vi "Parse Single Item.vi"(7 "Quoted String? (F)":bool, 11 "String In":string) -> (2 "Remaining":string, 3 "Item":string, 5 "JSON Item Type":T1=enum."null")   [LabVIEW 2020, in "JSON.lvlib"]
uses:
  JSON.lvlib
  JSON Item Type.ctl
  Unescape String.vi
  <vilib>/regexp/Match Regular Expression.xnode
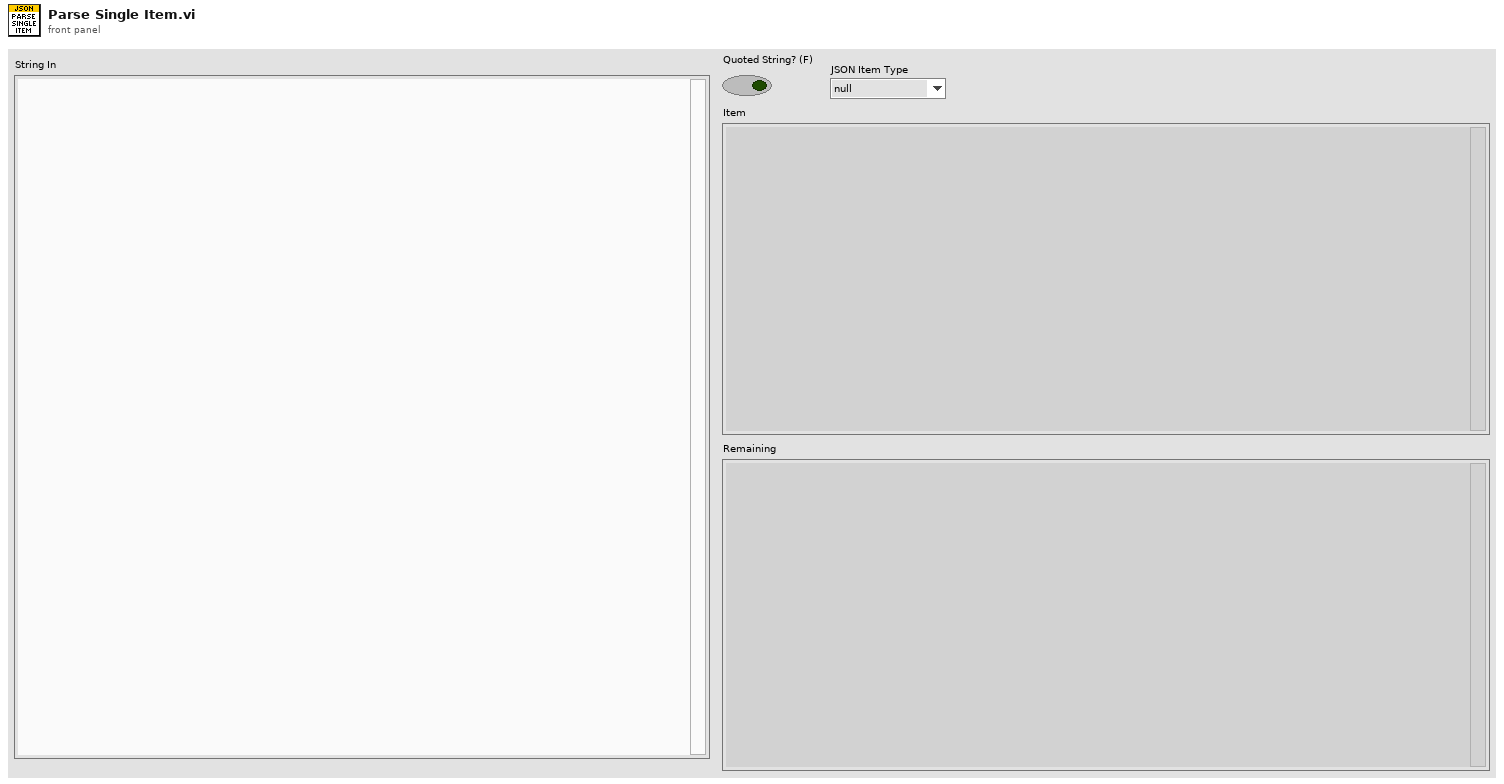
[diagram p1: front panel]
types:
  T1 = typedef "JSON.lvlib/JSON Item Type.ctl" = enum16{"unknown", "null", "Array", "Object", "String", "Number", "Boolean"}
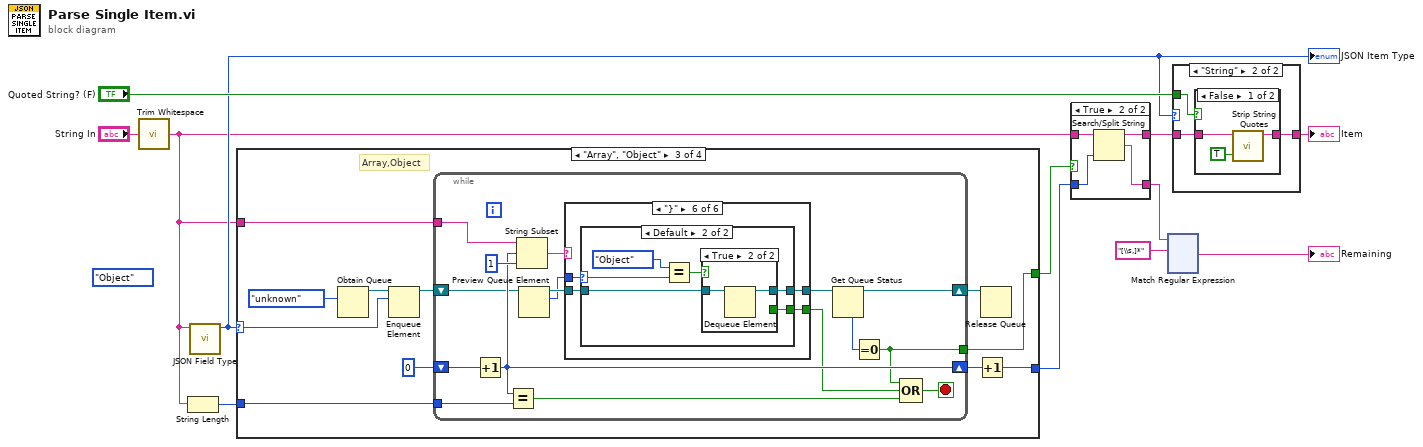
[diagram p0: block diagram]
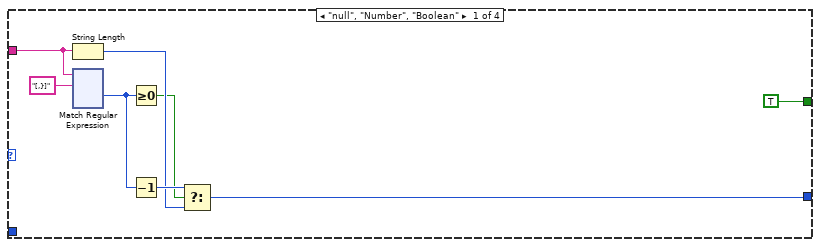
[diagram p4: hidden frame]
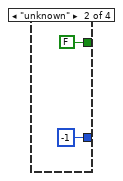
[diagram p5: hidden frame]
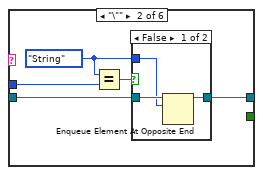
[diagram p7: hidden frame]
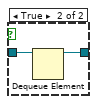
[diagram p8: hidden frame]
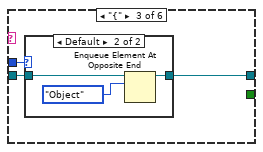
[diagram p9: hidden frame]
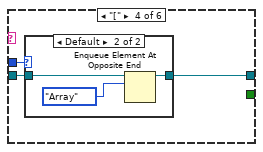
[diagram p11: hidden frame]
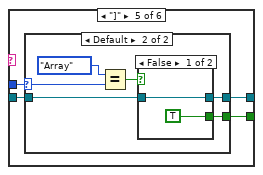
[diagram p13: hidden frame]
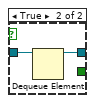
[diagram p15: hidden frame]
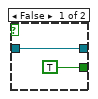
[diagram p17: hidden frame]
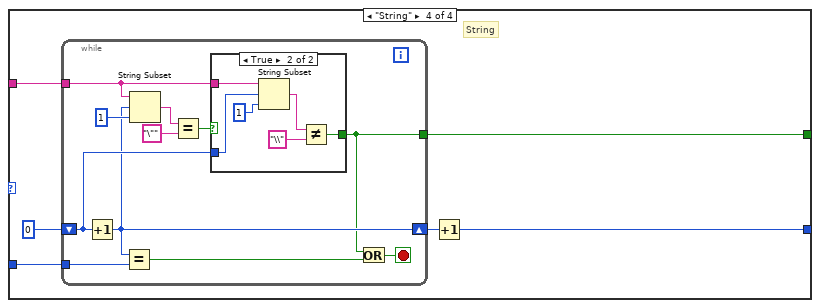
[diagram p18: hidden frame]
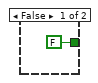
[diagram p19: hidden frame]
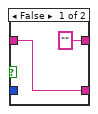
[diagram p20: hidden frame]
diagram:
  (unwired) JSON_Item_Type."Object" ("JSON Item Type")
  n1 = call <vilib>:"Trim Whitespace.vi"("string"="String In") -> ("trimmed string"=w1:string)  [unwired: 1 in]
  n2 = String Length(string=w1) -> (length=w11:i32)
  n3 = call "JSON Field Type.vi"("JSON String"=w1) -> ("JSON Item Type"=w2:T1)  [unwired: 10 in]
  "JSON Item Type" <- w2
  n4 = case shown="\"String\"" w2 {
    selector: w2 -> [_ _ w146 _]
    tunnel: w1 -> [w18 _ w144 w224]
    tunnel: w11 -> [_ _ w142 w223]
    tunnel: [w13 -1 w139 w219] -> w10
    tunnel: [TRUE FALSE w141 w220] -> w9
    frame "null", "Number", "Boolean" {
      n5 = String Length(string=w18) -> (length=w16:i32)
      n6 = xnode "Match Regular Expression"("input string"=w18, "regular expression"="[,}]") -> ("offset past match"=w19:i32)  [unwired: 4 in, 4 out]
      n7 = Greater Or Equal To 0?(x=w19) -> (x >= 0?=w15:bool)
      n8 = Decrement(x=w19) -> (x-1=w17:i32)
      n9 = Select(t=w17, s=w15, f=w16) -> (s? t:f=w13:i32)
    }
    frame "unknown" {
    }
    frame "Array", "Object" {
      # "Array,Object"
      n10 = Obtain Queue(element data type=JSON_Item_Type."unknown" ("JSON Item Type")) -> (queue out=w147:refnum<queue>)  [unwired: 4 in, 2 out]
      n11 = Enqueue Element(queue=w147, element=w146) -> (queue out=w145:refnum<queue>)  [unwired: 2 in, 2 out]
      n12 = while {
        shift-right: [w150] -> w138
        shift-left: w145 -> [w155]
        tunnel: w144 -> [w160]
        shift-right: [w156] -> w140
        shift-left: 0 -> [w158]
        tunnel: w142 -> [w163]
        tunnel: [w148] -> w141
        stop <- w161 stop-if-true
        n13 = Increment(x=w158) -> (x+1=w156:i32)
        n14 = Equal?(x=w156, y=w163) -> (x = y?=w162:bool)
        n15 = String Subset(string=w160, offset (0)=w156, length (rest)=1 ("length (rest)")) -> (substring=w157:string)
        n16 = Preview Queue Element(queue=w155) -> (queue out=w154:refnum<queue>, element=w153:T1)  [unwired: 2 in, 2 out]
        n17 = case shown="\"}\"" w157 {
          tunnel: w153 -> [_ w168 w175 w182 w190 w205]
          tunnel: w154 -> [w164 w167 w177 w184 w192 w207]
          tunnel: [w164 w166 w176 w183 w191 w206] -> w151
          tunnel: [_ _ _ _ w189 w204] -> w152
          frame Default {
          }
          frame "\"" {
            w165 = JSON_Item_Type."String" ("JSON Item Type")
            n18 = Equal?(x=w165, y=w168) -> (x = y?=w169:bool)
            n19 = case shown="False" w169 {
              tunnel: w167 -> [w172 w174]
              tunnel: [w171 w173] -> w166
              tunnel: w165 -> [w170 _]
              frame False {
                n20 = Enqueue Element At Opposite End(queue=w172, element=w170) -> (queue out=w171:refnum<queue>)  [unwired: 2 in, 2 out]
              }
              frame True {
                n21 = Dequeue Element(queue=w174) -> (queue out=w173:refnum<queue>)  [unwired: 2 in, 3 out]
              }
            }
          }
          frame "{" {
            n22 = case shown="Default" w175 {
              tunnel: w177 -> [w178 w181]
              tunnel: [w178 w180] -> w176
              frame "String" {
              }
              frame Default {
                n23 = Enqueue Element At Opposite End(queue=w181, element=JSON_Item_Type."Object" ("JSON Item Type")) -> (queue out=w180:refnum<queue>)  [unwired: 2 in, 2 out]
              }
            }
          }
          frame "[" {
            n24 = case shown="Default" w182 {
              tunnel: w184 -> [w185 w188]
              tunnel: [w185 w187] -> w183
              frame "String" {
              }
              frame Default {
                n25 = Enqueue Element At Opposite End(queue=w188, element=JSON_Item_Type."Array" ("JSON Item Type")) -> (queue out=w187:refnum<queue>)  [unwired: 2 in, 2 out]
              }
            }
          }
          frame "]" {
            n26 = case shown="Default" w190 {
              selector: w190 -> [_ w199]
              tunnel: w192 -> [w193 w197]
              tunnel: [w193 w196] -> w191
              tunnel: [_ w195] -> w189
              frame "String" {
              }
              frame Default {
                n27 = Equal?(x=JSON_Item_Type."Array" ("JSON Item Type"), y=w199) -> (x = y?=w198:bool)
                n28 = case shown="False" w198 {
                  tunnel: w197 -> [w201 w203]
                  tunnel: [w201 w202] -> w196
                  tunnel: [TRUE _] -> w195
                  frame False {
                  }
                  frame True {
                    n29 = Dequeue Element(queue=w203) -> (queue out=w202:refnum<queue>)  [unwired: 2 in, 3 out]
                  }
                }
              }
            }
          }
          frame "}" {
            n30 = case shown="Default" w205 {
              selector: w205 -> [_ w214]
              tunnel: w207 -> [w208 w212]
              tunnel: [w208 w211] -> w206
              tunnel: [_ w210] -> w204
              frame "String" {
              }
              frame Default {
                n31 = Equal?(x=JSON_Item_Type."Object" ("JSON Item Type"), y=w214) -> (x = y?=w213:bool)
                n32 = case shown="True" w213 {
                  tunnel: w212 -> [w216 w218]
                  tunnel: [w216 w217] -> w211
                  tunnel: [TRUE _] -> w210
                  frame False {
                  }
                  frame True {
                    n33 = Dequeue Element(queue=w218) -> (queue out=w217:refnum<queue>)  [unwired: 2 in, 3 out]
                  }
                }
              }
            }
          }
        }
        n34 = Get Queue Status(queue=w151) -> (queue out=w150:refnum<queue>, # elements in queue=w149:i32)  [unwired: 2 in, 6 out]
        n35 = Equal To 0?(x=w149) -> (x = 0?=w148:bool)
        n36 = Compound Arithmetic op=OR(w148, w152, w162) -> (w161:bool)
      }
      n37 = Increment(x=w140) -> (x+1=w139:i32)
      n38 = Release Queue(queue=w138) -> ()  [unwired: 2 in, 3 out]
    }
    frame "String" {
      # "String"
      n39 = while {
        tunnel: w224 -> [w229]
        shift-right: [w227] -> w221
        shift-left: 0 ("length (rest)") -> [w228]
        tunnel: w223 -> [w235]
        tunnel: [w226] -> w220
        stop <- w234 stop-if-true
        n40 = Increment(x=w228) -> (x+1=w227:i32)
        n41 = Equal?(x=w227, y=w235) -> (x = y?=w233:bool)
        n42 = String Subset(string=w229, offset (0)=w227, length (rest)=1 ("length (rest)")) -> (substring=w231:string)
        n43 = Equal?(x=w231, y="\"") -> (x = y?=w230:bool)
        n44 = case shown="False" w230 {
          tunnel: w229 -> [_ w241]
          tunnel: w228 -> [_ w240]
          tunnel: [FALSE w237] -> w226
          frame False {
          }
          frame True {
            n45 = String Subset(string=w241, offset (0)=w240, length (rest)=1 ("length (rest)")) -> (substring=w239:string)
            n46 = Not Equal?(x=w239, y="\\") -> (x != y?=w237:bool)
          }
        }
        n47 = Or(x=w226, y=w233) -> (x .or. y?=w234:bool)
      }
      n48 = Increment(x=w221) -> (x+1=w219:i32)
    }
  }
  n49 = case shown="True" w9 {
    tunnel: w1 -> [w244 w248]
    tunnel: w10 -> [_ w247]
    tunnel: ["" ("trimmed string") w246] -> w5
    tunnel: [w244 w245] -> w8
    frame False {
    }
    frame True {
      n50 = Search/Split String(string=w248, offset (0)=w247) -> (substring before match=w246:string, match + rest of string=w245:string)  [unwired: 1 in, 1 out]
    }
  }
  n51 = xnode "Match Regular Expression"("input string"=w8, "regular expression"="[\\s,]*") -> ("after match"=→"Remaining":string)  [unwired: 4 in, 4 out]
  n52 = case shown="\"String\"" w2 {
    tunnel: w5 -> [w249 w252]
    tunnel: [w249 w251] -> w4
    tunnel: "Quoted String? (F)" -> [_ w250]
    frame Default {
    }
    frame "String" {
      n53 = case shown="False" w250 {
        tunnel: w252 -> [w255 w256]
        tunnel: [w253 w256] -> w251
        frame False {
          n54 = call "Strip String Quotes.vi"("Skip Type Check? (F)"=TRUE, "JSON"=w255) -> ("Quotes Stripped"=w253:string)  [unwired: 9 in]
        }
        frame True {
        }
      }
    }
  }
  "Item" <- w4
